vi "TxChannel - Create Channel Configuration.vi"(7 "Add Port Channel":bool, 8 "error in (no error)":errorcluster, 11 "Parent Packet Ref":T1 format="%.0x") -> (0 "error out":errorcluster, 2 "Channel Config Ref":T1 format="%.0x")   [LabVIEW 2019, in "UDP-Custom-Device System Explorer.lvlib"]
uses:
  UDP-Custom-Device System Explorer.lvlib
  <vilib>/NI VeriStand/Custom Device API/Custom Device Item Ref.ctl
  <vilib>/NI VeriStand/Custom Device API/Custom Device Channel.ctl
  <vilib>/NI VeriStand/Custom Device API/Custom Device Channel Type.ctl
  Shared/Constants.vi
  <vilib>/NI VeriStand/Custom Device API/Custom Device API.lvlib
  Shared/UDP-Custom-Device Shared.lvlib
  Property Accessors/Shared Channel Accessors.lvlib
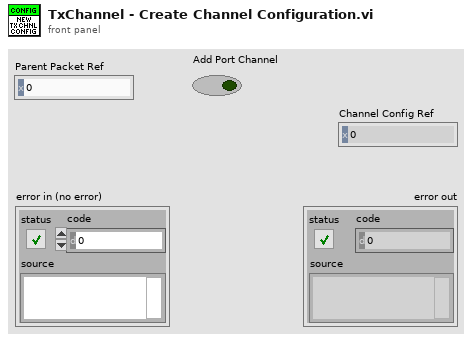
[diagram p1: front panel]
types:
  T1 = typedef "Custom Device API.lvlib/Custom Device Item Ref.ctl" = u64
  T2 = typedef "Custom Device API.lvlib/Custom Device Channel.ctl" = cluster{"Type":T3, "Units":string, "Default Value":dbl, "Faultable":bool, "Scalable":bool}
  T3 = typedef "Custom Device API.lvlib/Custom Device Channel Type.ctl" = enum16{"Input", "Output"}
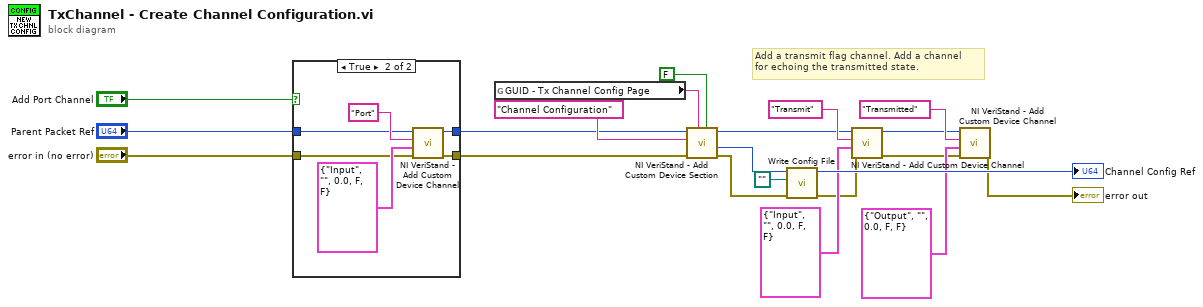
[diagram p0: block diagram]
diagram:
  # "Add a transmit flag channel. Add a channel\nfor echoing the transmitted state."
  n1 = case shown="True" "Add Port Channel" {
    tunnel: "error in (no error)" -> [w22 w27]
    tunnel: "Parent Packet Ref" -> [w23 w26]
    tunnel: [w23 w25] -> w8
    tunnel: [w22 w24] -> w7
    frame False {
    }
    frame True {
      n2 = call <vilib>:"NI VeriStand - Add Custom Device Channel.vi"("error in (no error)"=w27, "Channel"=T2 {"Type"=enum."Input", "Units"="", "Default Value"=0.0, "Faultable"=FALSE, "Scalable"=FALSE}, "Channel Name"="Port", "Parent Ref in"=w26) -> ("error out"=w24:errorcluster, "Parent Ref out"=w25:T1)  [unwired: 4 in, 2 out]
    }
  }
  n3 = global read "Constants.vi" "GUID - Tx Channel Config Page"() -> (w20:string)
  n4 = call <vilib>:"NI VeriStand - Add Custom Device Section.vi"("Highlight? (F)"=FALSE, "GUID (Default Section)"=w20, "error in (no error)"=w7, "Section Name"="Channel Configuration", "Parent Ref in"=w8) -> ("error out"=w15:errorcluster, "Section Ptr"=w16:T1, "Parent Ref out"=w12:T1)  [unwired: 3 in, 1 out]
  n5 = call "Write Config File.vi"("error in (no error)"=w15, "Config File"=path "", "Node Ptr"=w16) -> ("error out"=w11:errorcluster, "Node Ptr out"=→"Channel Config Ref":T1)  [unwired: 7 in]
  n6 = call <vilib>:"NI VeriStand - Add Custom Device Channel.vi"("error in (no error)"=w11, "Channel"=T2 {"Type"=enum."Input", "Units"="", "Default Value"=0.0, "Faultable"=FALSE, "Scalable"=FALSE}, "Channel Name"="Transmit", "Parent Ref in"=w12) -> ("error out"=w2:errorcluster, "Parent Ref out"=w3:T1)  [unwired: 4 in, 2 out]
  n7 = call <vilib>:"NI VeriStand - Add Custom Device Channel.vi"("error in (no error)"=w2, "Channel"=T2 {"Type"=enum."Output", "Units"="", "Default Value"=0.0, "Faultable"=FALSE, "Scalable"=FALSE}, "Channel Name"="Transmitted", "Parent Ref in"=w3) -> ("error out"=→"error out":errorcluster)  [unwired: 4 in, 3 out]
